vi "Header Create.vi"(10 "File Name":string, 11 "path File":path) -> (0 "error out":errorcluster, 3 "dup path":path)   [LabVIEW 2015]
uses:
  <vilib>/Utility/file.llb/Write Delimited Spreadsheet (string).vi
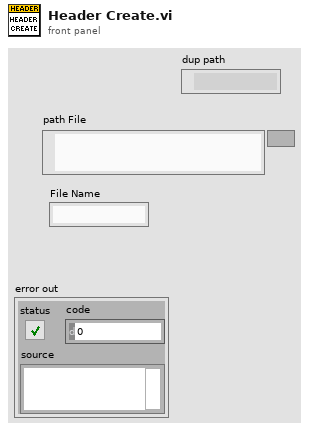
[diagram p1: front panel]
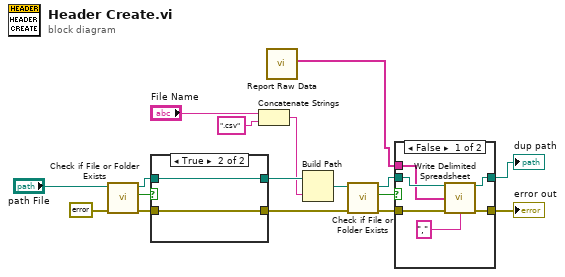
[diagram p0: block diagram]
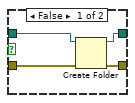
[diagram p3: hidden frame]
diagram:
  n1 = call <vilib>:"Check if File or Folder Exists.vi"("error in (no error)"=errorcluster {"status"=FALSE, "code"=0, "source"=""}, "path"="path File") -> ("error out"=w5:errorcluster, "file or folder exists?"=w7:bool, "dup path"=w6:path)  [unwired: 7 in]
  n2 = case shown="True" w7 {
    tunnel: [w21 w23] -> w11
    tunnel: [w20 w22] -> w8
    tunnel: w6 -> [w19 w23]
    tunnel: w5 -> [w18 w22]
    frame False {
      n3 = Create Folder(path (use dialog)=w19, error in=w18) -> (created path=w21:path, error out=w20:errorcluster)  [unwired: 1 in, 1 out]
    }
    frame True {
    }
  }
  n4 = Concatenate Strings("File Name", ".csv" ("string")) -> (w9:string)
  n5 = call "Report Raw Data.vi"() -> ("Header Name"=w1:string[])  [unwired: 11 in]
  n6 = Build Path(base path=w11, name or relative path=w9) -> (appended path=w14:path)
  n7 = call <vilib>:"Check if File or Folder Exists.vi"("error in (no error)"=w8, "path"=w14) -> ("error out"=w17:errorcluster, "file or folder exists?"=w15:bool, "dup path"=w16:path)  [unwired: 7 in]
  n8 = case shown="False" w15 {
    tunnel: w16 -> [w29 w31]
    tunnel: w17 -> [w28 w30]
    tunnel: [w26 w31] -> w13
    tunnel: [w25 w30] -> w12
    tunnel: w1 -> [w24 _]
    frame False {
      n9 = call-poly <vilib>:"Write Delimited Spreadsheet.vi"("file path (dialog if empty)"=w29, "1D data"=w24, "error in (no error)"=w28, "delimiter (\\t)"="," ("delimiter (\\t)")) -> ("new file path (Not A Path if cancelled)"=w26:path, "error out"=w25:errorcluster)  [unwired: 10 in]
    }
    frame True {
    }
  }
  "dup path" <- w13
  "error out" <- w12
